vi "Calc_Rel_Margin.vi"(0 "Max":sgl, 1 "Min":sgl) -> (14 "Rel_Margin":sgl)   [LabVIEW 2020]
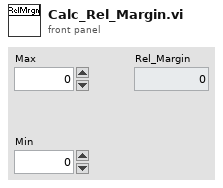
[diagram p1: front panel]
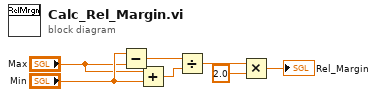
[diagram p0: block diagram]
diagram:
  n1 = Subtract(x="Min", y="Max") -> (x-y=w6:sgl)
  n2 = Add(x="Max", y="Min") -> (x+y=w7:sgl)
  n3 = Divide(x=w6, y=w7) -> (x/y=w3:sgl)
  n4 = Multiply(x=w3, y=sgl 2.0) -> (x*y=→"Rel_Margin":sgl)
